vi "BIG_DEMO_Queue.vi"() -> ()   [LabVIEW 2018]
uses:
  DataPacker/DataStructures/GEM_BANK_CLUSTER_typedef.ctl
  DataPacker/DataStructures/GEM_DATA_cluster_typedef.ctl
  <vilib>/Platform/TimedLoop/XDataNode/timing_clust.ctl
  <vilib>/Platform/TimedLoop/XDataNode/nitl_modes.ctl
  <vilib>/Platform/TimedLoop/XDataNode/wakeup.ctl
  0979d1a9-f879-4f92-9b98-5d0765c1d2d2.vi
  0979d1a9-f879-4f92-9b98-5d0765c1d2d2.vi/2aee1e73-4998-49f7-ad2d-0e099414d64d.vi
  <vilib>/platform/TimedLoop/XDataNode/XDataNode.xnode
  <vilib>/Platform/TimedLoop/XDataNode/XDNodeRunTimeDep.lvlib
panel:
  in  "MIDAS Sever Port":u16=12345
  in  "MIDAS Server":string="my_midas_server.domain"
  in  "stop":bool
  out "Run Stop Time":timestamp
  out "error out 2":errorcluster
  out "Run Start Time":timestamp
  out "error out":errorcluster
  in  "Override Max Event size (Data rate kb/s). MIDAS default=10":u32=100000000
  out "Get Run Status Error out":errorcluster
  out "Run Status":string
  out "Get RunNumber Error out":errorcluster
  in  "Period":i64=100
  in  "Override with Random Nums":bool
  in  "Category":string="CatchingTrap"
  in  "Number Of Vars In Category":i32=1
  in  "Number Of Categorys":i32=1
  out "RUNNO":i32
  in  "Double Array Var Name":string="A"
  in  "Event Limit":i32=2147483647
  out "# pending insert":i32
  out "# pending remove":i32
  out "# elements in queue":i32
  in  "Entries to log":i32=1
  in  "Temperature array":dbl[](array[numeric])=[0.1, 0.2, 0.3, 0.4, 0.5, 0.6, 0.7, 0.8, 0.9, 1.0]
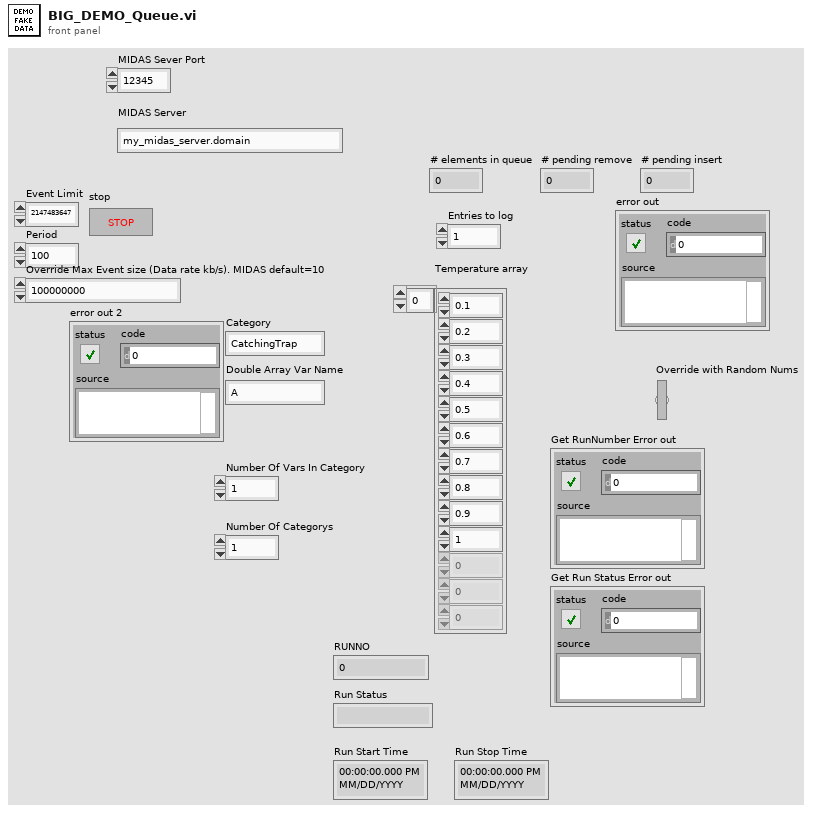
[diagram p1: front panel]
types:
  T1 = typedef "GEM_BANK_CLUSTER_typedef.ctl" = cluster{"Category":string, "Variable Name":string, "Equipment description":string, "History Settings":u16, "Period to update history plots":u16, "GEM_DATA Cluster":T2}
  T2 = typedef "GEM_DATA_cluster_typedef.ctl" = cluster{"DataType":string, "Formatted Data":u8[], "data byte order (Little Endian prefered)":enum16{"big-endian, network order", "native, host order", "little-endian"}}
  T3 = typedef "XDNodeRunTimeDep.lvlib/timing_clust.ctl" = cluster{"Expected End [f-1]":u64, "Actual End [f-1]":u64, "Finished Late? [f-1]":bool, "Expected End [i-1]":u64, "Actual End [i-1]":u64, "Finished Late? [i-1]":bool, "Expected Start [i]":u64, "Actual Start [i]":u64, "Expected Start [f]":u64, "Actual Start [f]":u64, "Source Name":string, "Structure Name":string, "Period":i64, "Deadline":i64, "Offset":i64, "Start":i64, "Priority":i32, "Timeout":i32, "Mode":T4, "Wakeup Reason":T5, "Error":errorcluster, "Source Type":string, "Secondary Source Type":string, "Global End Time":u64, "Global Start Time":u64, "Frame Duration":u64, "Iteration Duration":u64, "Assigned CPU":i32, "I/O Scan Engine Mode":u32}
  T4 = typedef "XDNodeRunTimeDep.lvlib/nitl_modes.ctl" = enum32{"No Change", "Process missed periods, maintain original phase", "Discard missed periods, maintain original phase", "Process missed periods, ignore original phase", "Discard missed periods, ignore original phase"}
  T5 = typedef "XDNodeRunTimeDep.lvlib/wakeup.ctl" = enum32{"Normal", "Aborted", "Asynchronous wakeup", "Timing source error", "Timed loop error", "Timeout"}
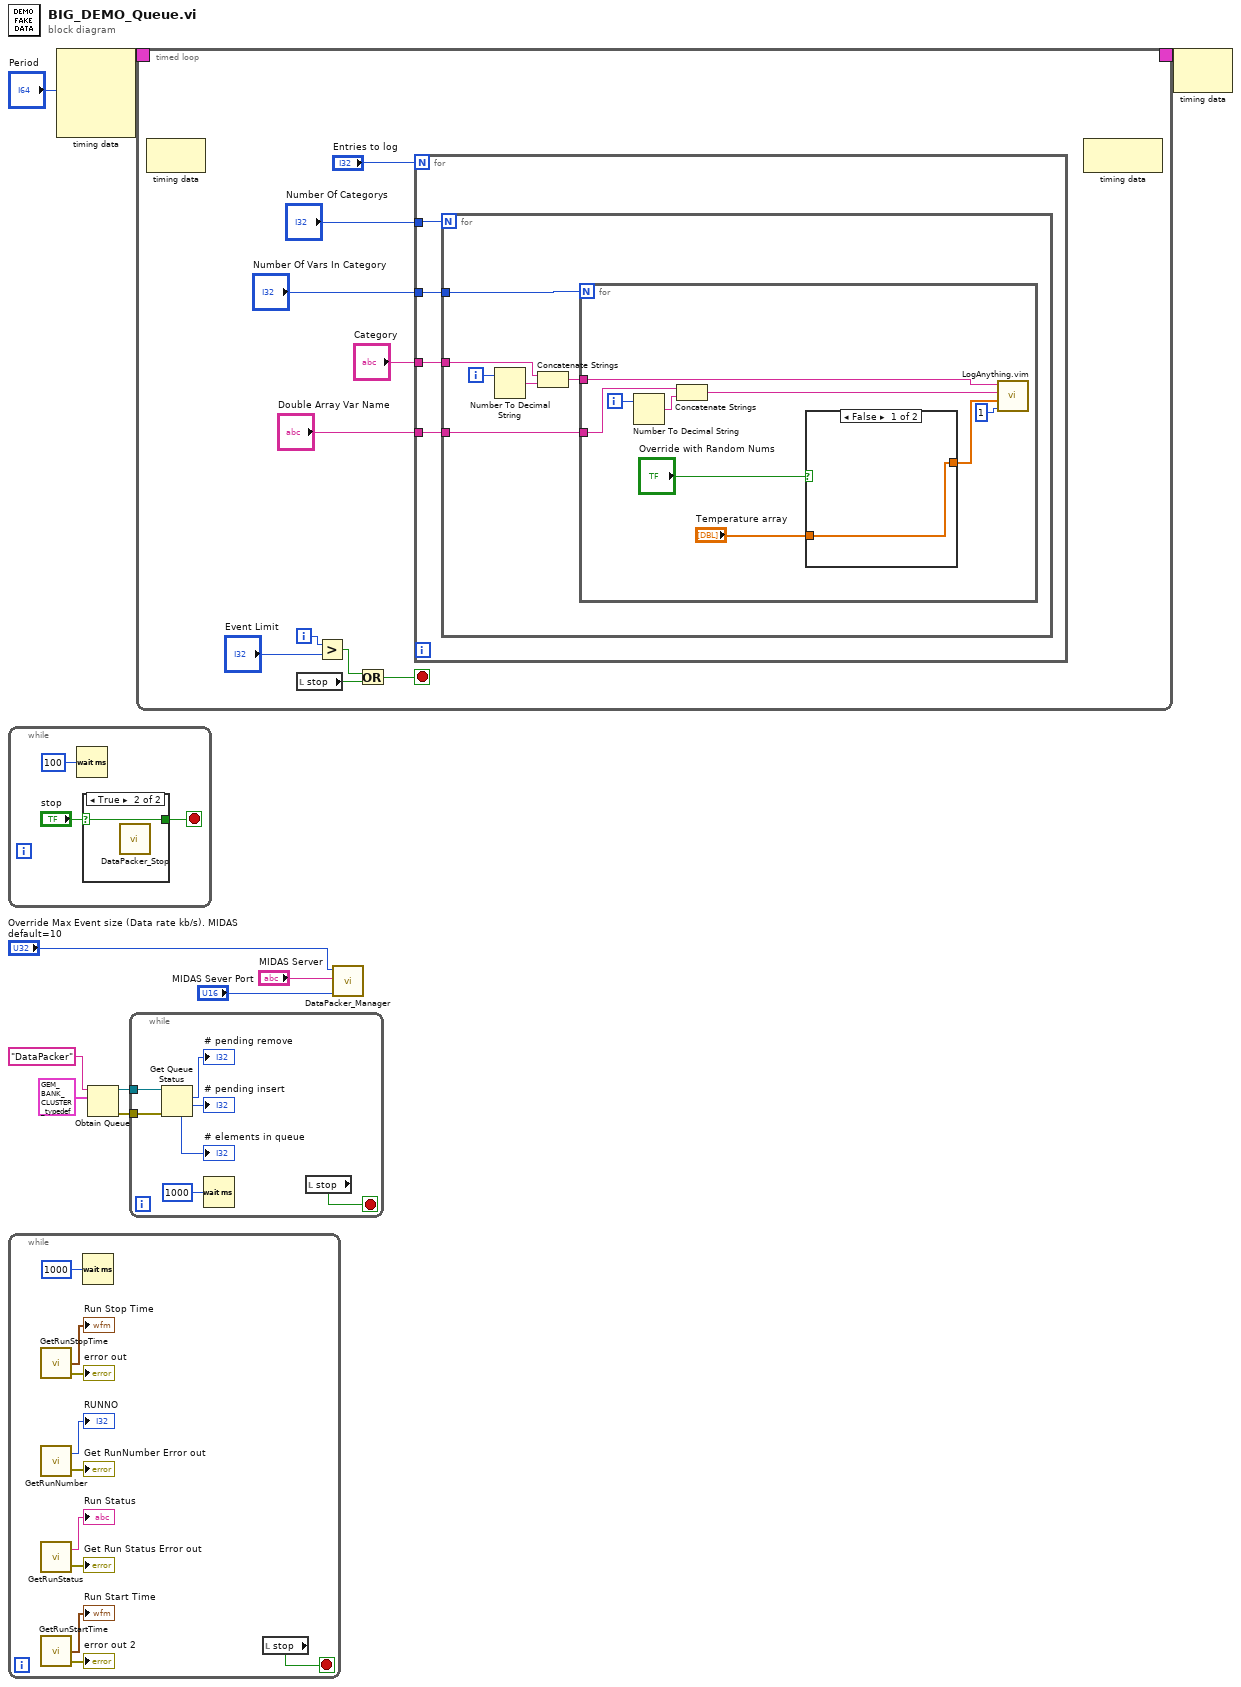
[diagram p0: block diagram]
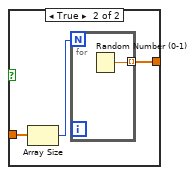
[diagram p3: hidden frame]
diagram:
  n1 = while {
    stop <- w11 stop-if-true
    n2 = Wait (ms)(milliseconds to wait=u32 100) -> ()  [unwired: 1 out]
    n3 = case shown="True" "stop" {
      selector: "stop" -> [w14 w15]
      tunnel: [w14 w15] -> w11
      frame False {
      }
      frame True {
        n4 = call "DataPacker_Stop.vi"() -> ()  [unwired: 12 in]
      }
    }
  }
  n5 = while {
    stop <- w16 stop-if-true
    n6 = call "GetRunStopTime.vi"() -> ("Run Stop Time"=→"Run Stop Time":timestamp, "error out"=→"error out":errorcluster)  [unwired: 2 in, 1 out]
    n7 = call "GetRunNumber.vi"() -> ("error out"=→"Get RunNumber Error out":errorcluster, "RunNumber"=→"RUNNO":i32)  [unwired: 2 in]
    n8 = call "GetRunStatus.vi"() -> ("error out"=→"Get Run Status Error out":errorcluster, "Run Status"=→"Run Status":string)  [unwired: 2 in]
    n9 = call "GetRunStartTime.vi"() -> ("Run Start Time"=→"Run Start Time":timestamp, "error out"=→"error out 2":errorcluster)  [unwired: 2 in, 1 out]
    n10 = Wait (ms)(milliseconds to wait=u32 1000) -> ()  [unwired: 1 out]
    n11 = local read "stop"() -> (w16:bool)
  }
  n12 = node-c288("Period") -> (w10:T3)  [unwired: 3 in]
  n13 = Obtain Queue(name (unnamed)="DataPacker", element data type=T1 {"Category"="", "Variable Name"="", "Equipment description"="", "History Settings"=0, "Period to update history plots"=0, "GEM_DATA Cluster"={"DataType"="", "Formatted Data"=[], "data byte order (Little Endian prefered)"=enum."big-endian, network order"}} ("output cluster")) -> (queue out=w6:refnum<queue>, error out=w3:errorcluster)  [unwired: 3 in, 1 out]
  n14 = while {
    tunnel: w6 -> [w32]
    tunnel: w3 -> [w26]
    stop <- w27 stop-if-true
    n15 = Get Queue Status(queue=w32, error in (no error)=w26) -> (# pending remove=→"# pending remove":i32, # pending insert=→"# pending insert":i32, # elements in queue=→"# elements in queue":i32)  [unwired: 1 in, 5 out]
    n16 = Wait (ms)(milliseconds to wait=u32 1000) -> ()  [unwired: 1 out]
    n17 = local read "stop"() -> (w27:bool)
  }
  n18 = timed-loop {
    timing: w10 -> [_]
    timing-out: [_] -> w9
    i -> [w41]
    stop <- w34 stop-if-true
    n19 = node-c288() -> ()  [unwired: 1 in, 1 out]
    n20 = local read "stop"() -> (w33:bool)
    n21 = Greater?(x=w41, y="Event Limit") -> (0:w35:bool)
    n22 = Or(x=w35, y=w33) -> (x .or. y?=w34:bool)
    n23 = for {
      N: "Entries to log" -> [_]
      tunnel: "Number Of Categorys" -> [w44]
      tunnel: "Number Of Vars In Category" -> [w45]
      tunnel: "Double Array Var Name" -> [w46]
      tunnel: "Category" -> [w43]
      n24 = for {
        N: w44 -> [_]
        tunnel: w45 -> [w52]
        tunnel: w46 -> [w51]
        tunnel: w43 -> [w50]
        i -> [w48]
        n25 = Number To Decimal String(number=w48) -> (decimal integer string=w49:string)  [unwired: 1 in]
        n26 = Concatenate Strings(w50, w49) -> (w47:string)
        n27 = for {
          N: w52 -> [_]
          tunnel: w51 -> [w60]
          tunnel: w47 -> [w53]
          i -> [w59]
          n28 = Number To Decimal String(number=w59) -> (decimal integer string=w61:string)  [unwired: 1 in]
          n29 = Concatenate Strings(w60, w61) -> (w54:string)
          n30 = case shown="False" "Override with Random Nums" {
            tunnel: "Temperature array" -> [w62 w65]
            tunnel: [w62 w63] -> w56
            frame False {
            }
            frame True {
              n31 = Array Size(array=w65) -> (size(s)=w64:i32)
              n32 = for {
                N: w64 -> [_]
                tunnel: [w66] -> w63 mode=indexing
                n33 = Random Number (0-1)() -> (number: 0 to 1=w66:dbl)
              }
            }
          }
          n34 = call "LogAnything.vim"("Period to update history plots (seconds)\nUnset (65535) = Use MIDAS default in ODB\n0 = Record but do not put in histories"=1 ("Rate to update history plots"), "Array"=w56, "Var Name"=w54, "Category"=w53) -> ()  [unwired: 3 in, 1 out]
        }
      }
    }
    n35 = node-c288() -> ()  [unwired: 1 in, 1 out]
  }
  n36 = call "DataPacker_Manager.vi"("MIDAS Sever Port"="MIDAS Sever Port", "MIDAS Server"="MIDAS Server", "Override Max Event size (Data rate kb/s). Use MIDAS Default = 0"="Override Max Event size (Data rate kb/s). MIDAS default=10") -> ()  [unwired: 9 in]
  n37 = node-c288(w9) -> ()  [unwired: 1 out]
